vi "Agilent N934X Series Read Demodulation Measurement.vi"() -> ()   [LabVIEW 2022 SP3]
doc: "This example shows how to read the measurement data in demodulation mode.\n\n<B>Note:</B> \n\n(1) This example is only applicable for N9322C."
uses:
  <instrlib>/Agilent N934X Series/Agilent N934X Series.lvlib
panel:
  in  "Measurement Mode (0: Off)":i32(ring)=7 items=["Off", "Channel Power Measurement", "Adjacent Channel Power Ratio Measurement", "Occupied Bandwidth Measurement", "Spectrum Monitor", "Spectrum Emission Mask", "Channel Scanner", "AM Measurement", "ASK Measurement", "FM Measurement", "FSK Measurement"]
  out "THD":dbl[](array[numeric])
  in  "Detector Type (0: Positive Peak)":i32(ring) items=["Positive Peak", "Negative Peak", "Average Peak", "RMS"]
  in  "Carrier Frequency Step (1E+8 Hz)":dbl=100000000.0
  in  "External Gain (0 dB)":dbl
  in  "Carrier Frequency (2.5E+6 Hz)":dbl=2500000.0
  in  "Measurement Type (0: Spectrum Analyzer)":i32(ring)=3 items=["Spectrum Analyzer", "Tracking Generator", "Power Meter", "Modulation Analyzer", "Reflection Measurement"]
  out "SINAD":dbl[](array[numeric])
  out "Modulation Rate":dbl[](array[numeric])
  out "Carrier Frequency Offset":dbl[](array[numeric])
  out "AM Depth":dbl[](array[numeric])
  out "Carrier Power":dbl[](array[numeric])
  in  "Measurement Duration (10 s)":u16=10
  in  "VISA resource name":refnum<visa-resource-name>
  # "(c) 2012-2025 National Instruments.  ALL RIGHTS RESERVED."
  # "Data Format:\nArray[0] : Current Value\nArray[1] : MAX Value\nArray[2] : MIN Value"
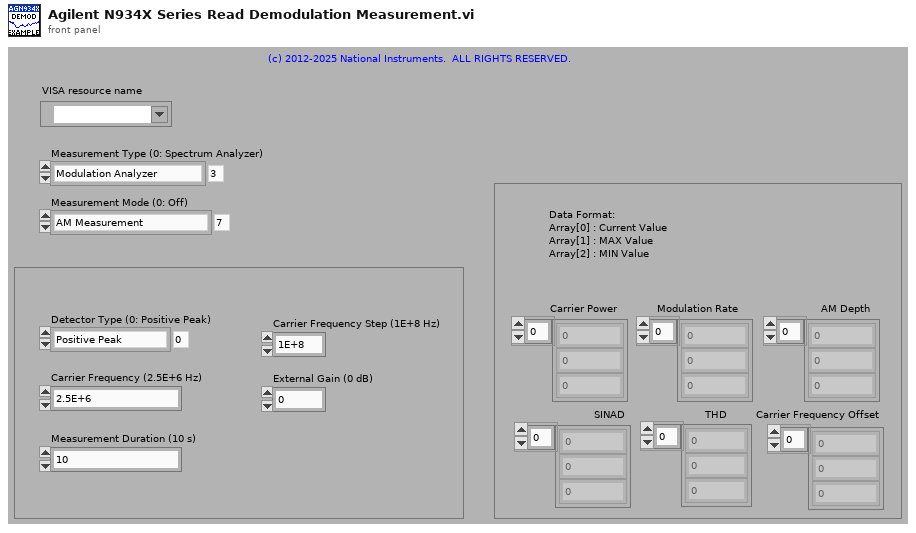
[diagram p1: front panel]
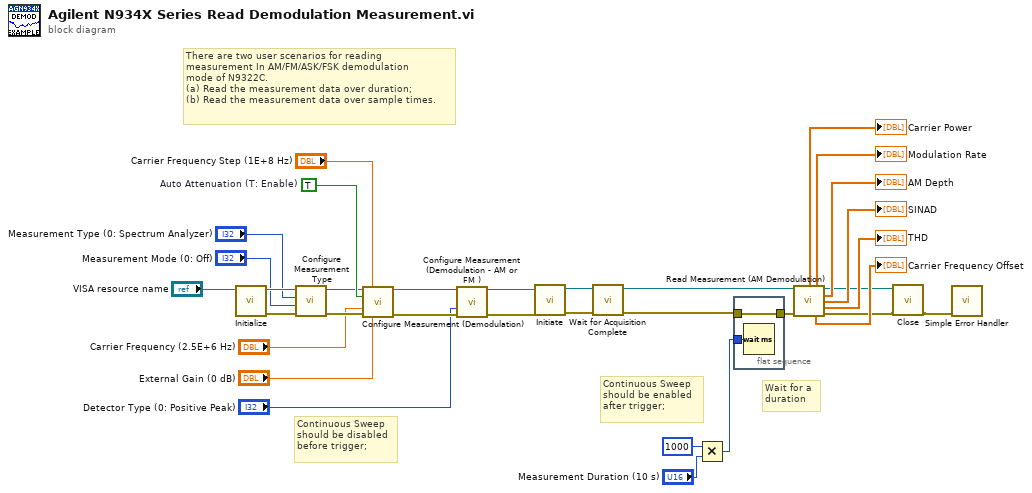
[diagram p0: block diagram]
diagram:
  w24 = TRUE  # Auto Attenuation (T: Enable)
  # "Wait for a \nduration"
  # "Continuous Sweep\nshould be enabled\nafter trigger;"
  # "Continuous Sweep\nshould be disabled\nbefore trigger;"
  # "There are two user scenarios for reading \nmeasurement In AM/FM/ASK/FSK demodulation \nmode of N9322C.\n(a) Read the measurement data over duration;\n(b) Read the measurement data over sample times."
  n1 = call <instrlib>:"Initialize.vi"("VISA resource name"="VISA resource name") -> ("error out"=w28:errorcluster, "VISA resource name out"=w29:refnum<visa-resource-name>)  [unwired: 9 in]
  n2 = call <instrlib>:"Configure Measurement Type.vi"("error in (no error)"=w28, "Measurement Mode (0: Off)"="Measurement Mode (0: Off)", "Measurement Type (0: Spectrum Analyzer)"="Measurement Type (0: Spectrum Analyzer)", "VISA resource name"=w29) -> ("error out"=w22:errorcluster, "VISA resource name out"=w23:refnum<visa-resource-name>)  [unwired: 6 in]
  n3 = call <instrlib>:"Configure Measurement (Demodulation).vi"("VISA resource name"=w23, "Carrier Frequency Step (1E+8 Hz)"="Carrier Frequency Step (1E+8 Hz)", "Auto Carrier Frequency (F: Disable)"=w24, "Carrier Frequency (2.5E+6 Hz)"="Carrier Frequency (2.5E+6 Hz)", "error in (no error)"=w22, "External Gain (0 dB)"="External Gain (0 dB)") -> ("VISA resource name out"=w19:refnum<visa-resource-name>, "error out"=w18:errorcluster)  [unwired: 8 in]
  n4 = call <instrlib>:"Configure Measurement (Demodulation - AM or FM ).vi"("VISA resource name"=w19, "Detector Type (0: Positive Peak)"="Detector Type (0: Positive Peak)", "error in (no error)"=w18) -> ("VISA resource name out"=w16:refnum<visa-resource-name>, "error out"=w15:errorcluster)  [unwired: 11 in]
  n5 = call <instrlib>:"Initiate.vi"("error in (no error)"=w15, "VISA resource name"=w16) -> ("error out"=w25:errorcluster, "VISA resource name out"=w26:refnum<visa-resource-name>)  [unwired: 8 in]
  n6 = call <instrlib>:"Wait for Acquisition Complete.vi"("error in (no error)"=w25, "VISA resource name"=w26) -> ("error out"=w14:errorcluster, "VISA resource name out"=w3:refnum<visa-resource-name>)  [unwired: 8 in]
  n7 = Multiply(x=u32 1000, y="Measurement Duration (10 s)") -> (x*y=w31:u32)
  n8 = flat-sequence {
    tunnel: w31 -> [w35]
    tunnel: [w34] -> w13
    tunnel: w14 -> [w34]
    frame #0 {
      n9 = Wait (ms)(milliseconds to wait=w35) -> ()  [unwired: 1 out]
    }
  }
  n10 = call <instrlib>:"Read Measurement (AM Demodulation).vi"("VISA resource name"=w3, "error in (no error)"=w13) -> ("Carrier Power (dBm)"=→"Carrier Power":dbl[], "Modulation Rate (Hz)"=→"Modulation Rate":dbl[], "VISA resource name out"=w6:refnum<visa-resource-name>, "AM Depth (%)"=→"AM Depth":dbl[], "SINAD (dB)"=→"SINAD":dbl[], "THD (dB)"=→"THD":dbl[], "Carrier Frequency Offset (Hz)"=→"Carrier Frequency Offset":dbl[], "error out"=w5:errorcluster)  [unwired: 6 in]
  n11 = call <instrlib>:"Close.vi"("error in (no error)"=w5, "VISA resource name"=w6) -> ("error out"=w4:errorcluster)  [unwired: 9 in]
  n12 = call <vilib>:"Simple Error Handler.vi"("error in (no error)"=w4) -> ()  [unwired: 1 in, 8 out]
